vi "Convert To HTML.vi"(8 "error in (no error)":errorcluster, 10 "HTML File Path":path, 11 "Document in":refnum<class "Document.lvclass">) -> (0 "error out":errorcluster, 3 "Document out":refnum<class "Document.lvclass">)   [LabVIEW 2017, in "LabVIEW NPOI.lvlib" / "Document.lvclass"]
uses:
  Document.lvclass
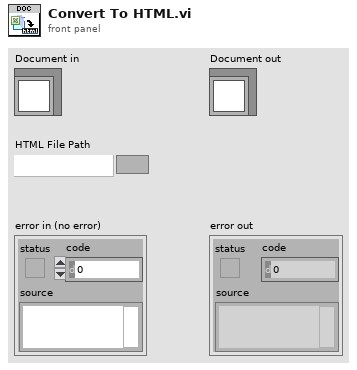
[diagram p1: front panel]
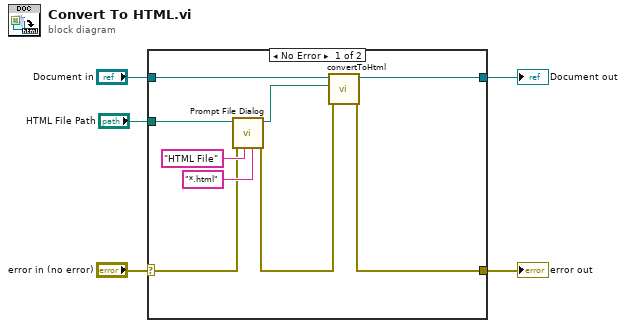
[diagram p0: block diagram]
diagram:
  n1 = case shown="No Error" "error in (no error)" {
    selector: "error in (no error)" -> [w11 w16]
    tunnel: "HTML File Path" -> [w14 _]
    tunnel: [w7 w16] -> w3
    tunnel: "Document in" -> [w10 w15]
    tunnel: [w9 w15] -> w1
    frame No Error {
      n2 = call "Prompt File Dialog.vi"("pattern (all files)"="*.html", "pattern label"="HTML File", "error in"=w11, "File Path"=w14) -> ("error out"=w8:errorcluster, "selected path"=w6:path)  [unwired: 6 in]
      n3 = call-dynamic "convertToHtml.vi"("error in (no error)"=w8, "HTML File Path"=w6, "Document in"=w10) -> ("error out"=w7:errorcluster, "Document out"=w9:refnum<class "Document.lvclass">)  [unwired: 7 in]
    }
    frame Error {
    }
  }
  "error out" <- w3
  "Document out" <- w1
